vi "Is Buffer Full?.vi"(8 "Triggered?":bool, 9 "Buffer in Points":dbl, 10 "Index location":dbl, 11 "output waveform":waveform(dbl)) -> (3 "Buffer Full?":bool)   [LabVIEW 2014]
panel:
  # "Is Buffer Full? VI"
  # "Inputs"
  # "Outputs"
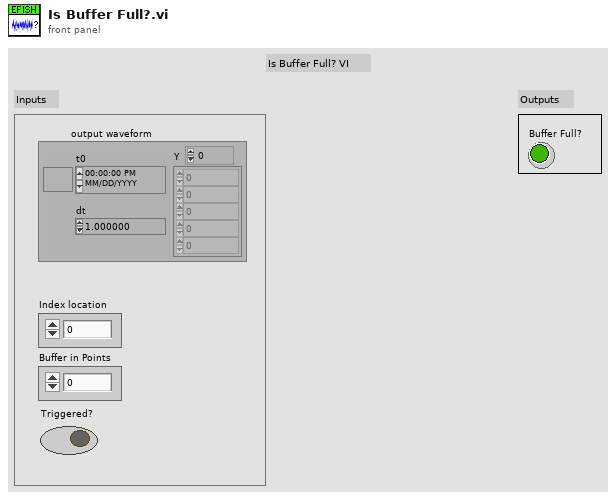
[diagram p1: front panel]
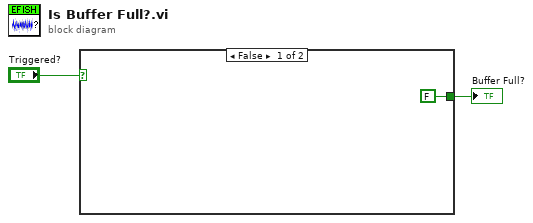
[diagram p0: block diagram]
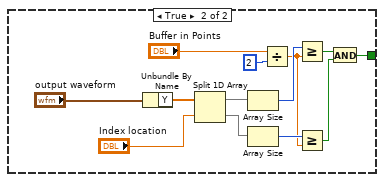
[diagram p2: hidden frame]
diagram:
  n1 = case shown="False" "Triggered?" {
    tunnel: [FALSE w4] -> w2
    frame False {
    }
    frame True {
      n2 = Unbundle By Name("output waveform") -> ("Y"=w13:dbl[])
      n3 = Split 1D Array(array=w13, index="Index location") -> (first subarray=w11:dbl[], second subarray=w10:dbl[])
      n4 = Array Size(array=w11) -> (size(s)=w9:i32)
      n5 = Array Size(array=w10) -> (size(s)=w8:i32)
      n6 = Divide(x="Buffer in Points", y=2) -> (x/y=w7:dbl)
      n7 = Greater Or Equal?(x=w9, y=w7) -> (x >= y?=w6:bool)
      n8 = Greater Or Equal?(x=w8, y=w7) -> (x >= y?=w5:bool)
      n9 = And(x=w6, y=w5) -> (x .and. y?=w4:bool)
    }
  }
  "Buffer Full?" <- w2
